vi "ADCReq.vi"(0 "aDATA":u8[](array[numeric]), 2 "ch":u8, 4 "Gain":dbl, 5 "Rsense":dbl) -> (12 "ADC Unit":dbl, 14 "ADC UnitT1":dbl, 15 "ADC UnitT2":dbl, 16 "ADC UnitT3":dbl, 17 "ADC UnitT4":dbl)   [LabVIEW 2017]
panel:
  # "ch1 = 0\nch2=1\nch3=2\nch4=3"
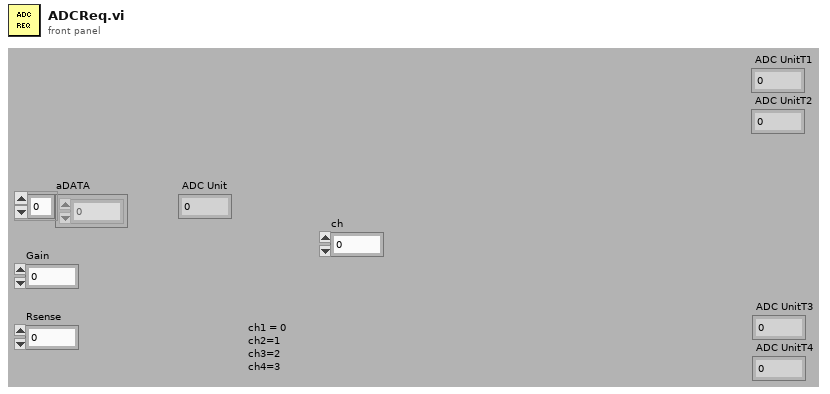
[diagram p1: front panel]
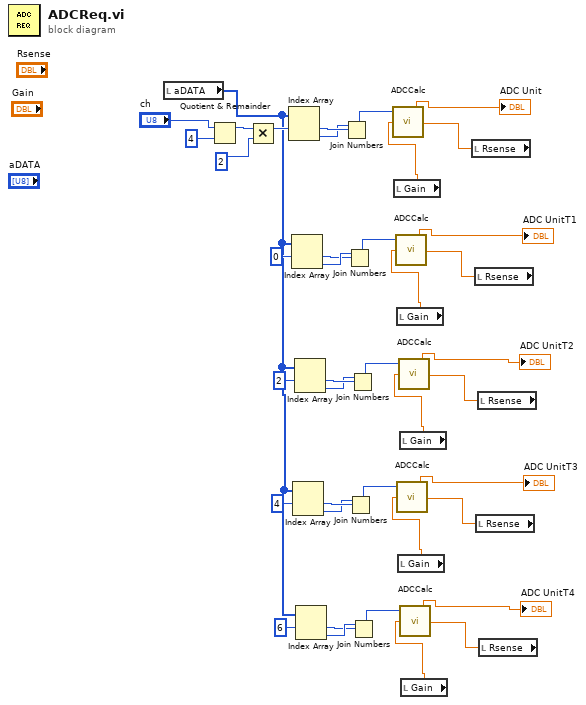
[diagram p0: block diagram]
diagram:
  n1 = local read "aDATA"() -> (w1:u8[])
  n2 = Quotient & Remainder(x="ch", y=u8 4) -> (x-y*floor(x/y)=w34:u8)  [unwired: 1 out]
  n3 = Multiply(x=w34, y=u8 2) -> (x*y=w37:u8)
  n4 = Index Array(array=w1, index #1=w37) -> (element #1=w40:u8, element #2=w39:u8)  [unwired: 1 in]
  n5 = Index Array(array=w1, index #1=0 ("index")) -> (element #1=w25:u8, element #2=w26:u8)  [unwired: 1 in]
  n6 = Index Array(array=w1, index #1=4 ("index")) -> (element #1=w6:u8, element #2=w5:u8)  [unwired: 1 in]
  n7 = Index Array(array=w1, index #1=2 ("index")) -> (element #1=w24:u8, element #2=w23:u8)  [unwired: 1 in]
  n8 = Index Array(array=w1, index #1=6 ("index")) -> (element #1=w7:u8, element #2=w8:u8)  [unwired: 1 in]
  n9 = Join Numbers(hi=w39, lo=w40) -> ((hi.lo)=w38:u16)
  n10 = Join Numbers(hi=w26, lo=w25) -> ((hi.lo)=w27:u16)
  n11 = Join Numbers(hi=w5, lo=w6) -> ((hi.lo)=w4:u16)
  n12 = Join Numbers(hi=w23, lo=w24) -> ((hi.lo)=w22:u16)
  n13 = Join Numbers(hi=w8, lo=w7) -> ((hi.lo)=w9:u16)
  n14 = local read "Gain"() -> (w32:dbl)
  n15 = local read "Gain"() -> (w29:dbl)
  n16 = local read "Gain"() -> (w2:dbl)
  n17 = local read "Gain"() -> (w20:dbl)
  n18 = local read "Gain"() -> (w11:dbl)
  n19 = local read "Rsense"() -> (w33:dbl)
  n20 = call "ADCCalc.vi"("Rsense"=w33, "Gain"=w32, "DATA"=w38) -> ("NumOut"=→"ADC Unit":dbl)
  n21 = local read "Rsense"() -> (w28:dbl)
  n22 = call "ADCCalc.vi"("Rsense"=w28, "Gain"=w29, "DATA"=w27) -> ("NumOut"=→"ADC UnitT1":dbl)
  n23 = local read "Rsense"() -> (w3:dbl)
  n24 = call "ADCCalc.vi"("Rsense"=w3, "Gain"=w2, "DATA"=w4) -> ("NumOut"=→"ADC UnitT3":dbl)
  n25 = local read "Rsense"() -> (w21:dbl)
  n26 = call "ADCCalc.vi"("Rsense"=w21, "Gain"=w20, "DATA"=w22) -> ("NumOut"=→"ADC UnitT2":dbl)
  n27 = local read "Rsense"() -> (w10:dbl)
  n28 = call "ADCCalc.vi"("Rsense"=w10, "Gain"=w11, "DATA"=w9) -> ("NumOut"=→"ADC UnitT4":dbl)
